vi "TimingToPoints.vi"(10 "Device":T1, 11 "Timing":T2 {"Pre-trigger length" format="%#_4p"; "Record length" format="%#_6p"; "Data rate" format="%#_6p"}) -> (0 "Pre-trigger position, %":dbl, 1 "Pre-trigger points":i64, 2 "Total points":i64, 3 "Actual Rate, Hz":dbl)   [LabVIEW 2015]
uses:
  Controls/Timing Element.ctl
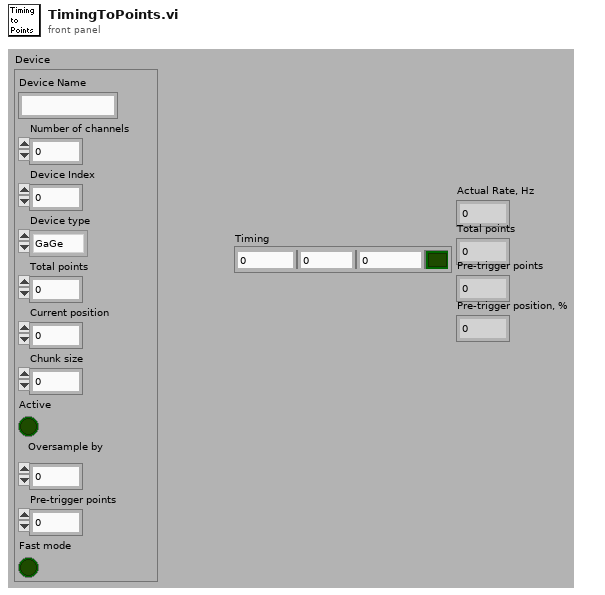
[diagram p1: front panel]
types:
  T1 = cluster{"Device Name":string, "Number of channels":i32, "Device Index":i32, "Device type":enum16{"GaGe", "NI-DAQ", "NI-Scope", "CAMAC", "VXI-1433", "VXI-1437"}, "Total points":i64, "Current position":i64, "Chunk size":i64, "Active":bool, "Oversample by":i32, "Pre-trigger points":i64, "Fast mode":bool}
  T2 = typedef "Timing Element.ctl" = cluster{"Data rate":dbl, "Record length":dbl, "Pre-trigger length":dbl, "Ext. clock":bool}
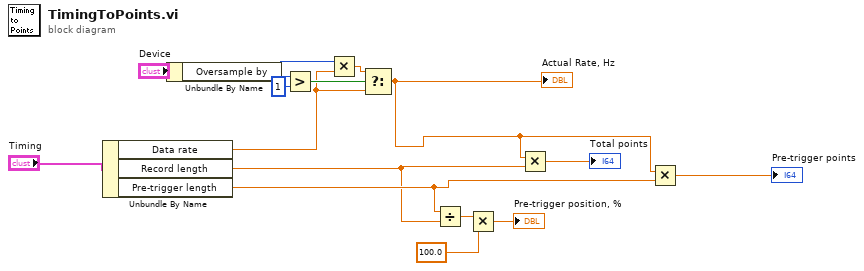
[diagram p0: block diagram]
diagram:
  n1 = Unbundle By Name("Timing") -> ("Data rate"=w3:dbl, "Record length"=w8:dbl, "Pre-trigger length"=w9:dbl)
  n2 = Unbundle By Name("Device") -> ("Oversample by"=w2:i32)
  n3 = Greater?(x=w2, y=1) -> (0:w5:bool)
  n4 = Multiply(x=w2, y=w3) -> (x*y=w4:dbl)
  n5 = Select(t=w4, s=w5, f=w3) -> (s? t:f=w1:dbl)
  "Actual Rate, Hz" <- w1
  n6 = Divide(x=w9, y=w8) -> (x/y=w12:dbl)
  n7 = Multiply(x=w12, y=100.0) -> (x*y=→"Pre-trigger position, %":dbl)
  n8 = Multiply(x=w1, y=w8) -> (x*y=→"Total points":dbl)
  n9 = Multiply(x=w1, y=w9) -> (x*y=→"Pre-trigger points":dbl)
